vi "local.Read Dev.Chassis.vi"(8 "error in (no error)":errorcluster, 11 "SLSC Local in":refnum<class "SLSC Interface.lvclass">) -> (0 "error out":errorcluster, 2 "Dev.Chassis":refnum<k21>, 3 "SLSC Local out":refnum<class "SLSC Interface.lvclass">)   [LabVIEW 2016, in "SLSC Interface.lvclass"]
uses:
  SLSC Interface Class/SLSC Interface.lvclass
  SLSC Interface Class/Read session.vi
  <resource>/objmgr/slsc.rc
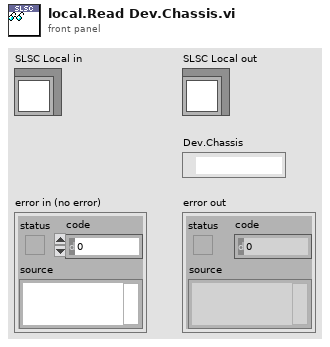
[diagram p1: front panel]
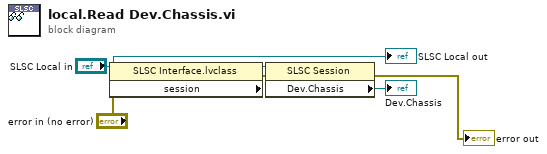
[diagram p0: block diagram]
diagram:
  n1 = property class="SLSC Interface.lvclass"(reference="SLSC Local in", error in="error in (no error)") -> (error out=w5:errorcluster, "session"=w6:refnum<k21>)  [unwired: 1 out]
  n2 = property class="SLSC Session"(reference=w6, error in=w5) -> (error out=→"error out":errorcluster, "Dev.Chassis"=→"Dev.Chassis":refnum<k21>)  [unwired: 1 out]
  "SLSC Local out" <- "SLSC Local in"
